vi "CLD 15 Address Parsing SubVI.vi"(8 "Fehler (Eingang)":errorcluster, 10 "Daten-String (Eingang)":string, 11 "Datenstruktur der CSV-Datei (Eingang)":T1) -> (0 "Fehler (Ausgang)":errorcluster, 3 "Datenstruktur der CSV-Datei (Ausgang)":T1)   [LabVIEW 2009]
doc: "CLD 15 - Analyseroutine für den Adress-String in CLD 15. Dieser String enthält auch den Rabatt in Prozent. Die Preise und der Schwellwert für eine Großbestellung werden der Spezifikation entnommen.\n\nDie Datenformate werden der Spezifikation als freie Beschriftungen entnommen, um zu vermeiden, dass sie während der Programmierung erneut geprüft werden."
uses:
  CLD 15 CSV file data structure.ctl
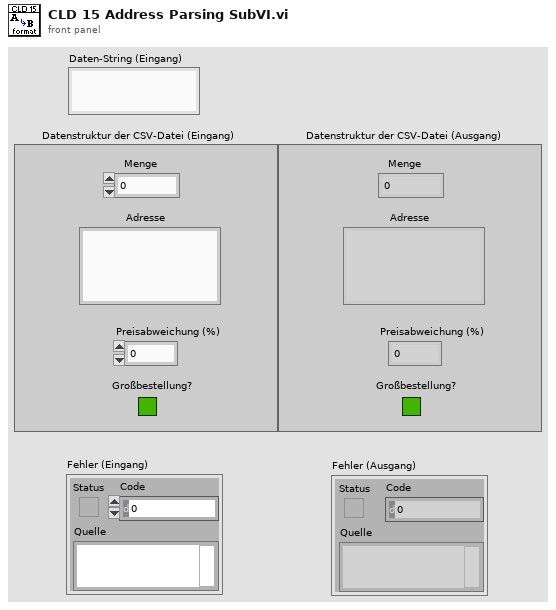
[diagram p1: front panel]
types:
  T1 = typedef "CLD 15 CSV file data structure.ctl" = cluster{"Menge":i32, "Adresse":string, "Preisabweichung (%)":dbl, "Großbestellung?":bool}
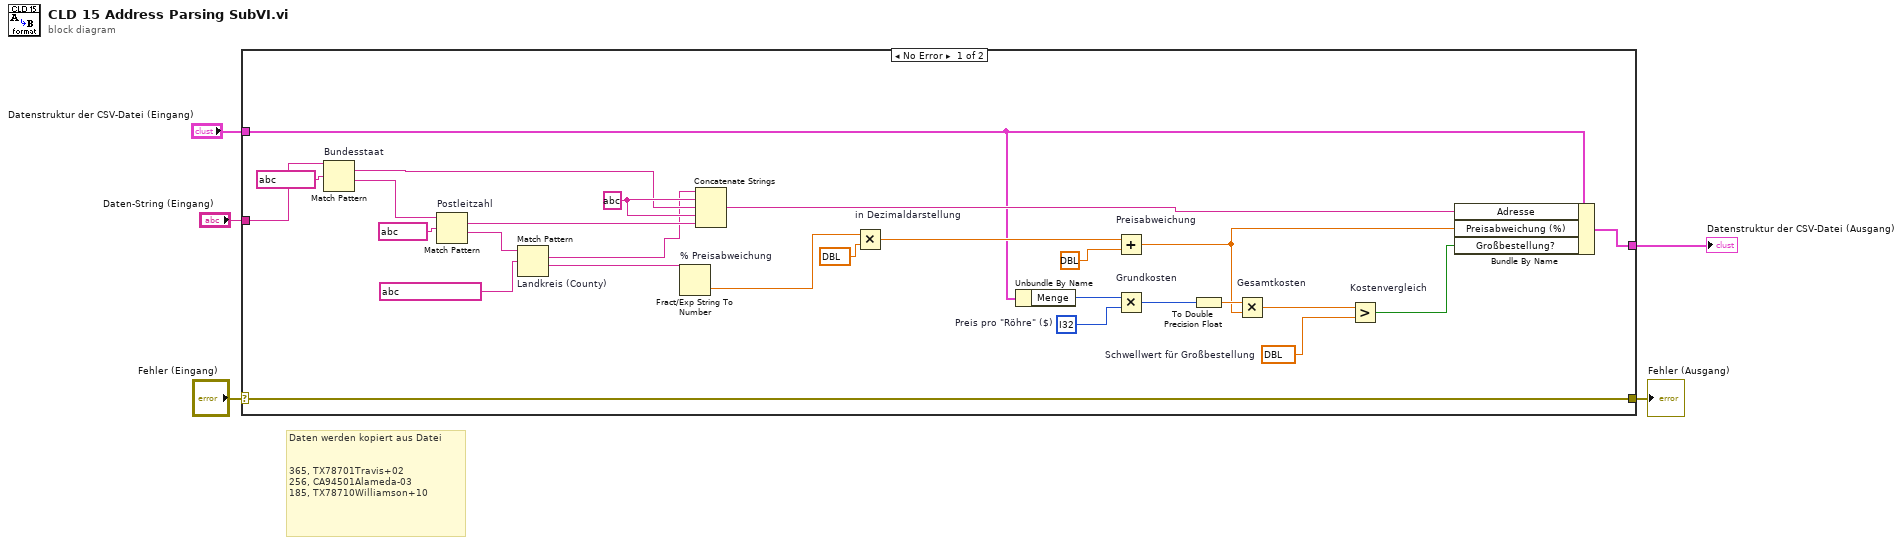
[diagram p0: block diagram]
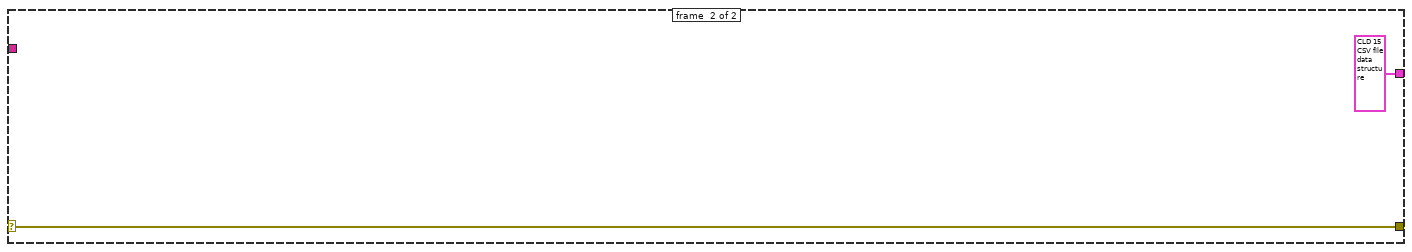
[diagram p2: hidden frame]
diagram:
  # "Daten werden kopiert aus Datei\n\n\n365,\tTX78701Travis+02\n256,\tCA94501Alameda-03\n185,\tTX78710Williamson+10"
  n1 = case shown="No Error" "Fehler (Eingang)" {
    selector: "Fehler (Eingang)" -> [w7 w34]
    tunnel: [w32 T1 ? ("Datenstruktur der CSV-Datei (Eingang)")] -> w5
    tunnel: "Daten-String (Eingang)" -> [w31 _]
    tunnel: [w7 w34] -> w2
    tunnel: "Datenstruktur der CSV-Datei (Eingang)" -> [w6 _]
    frame #0 {
      w14 = dbl ?  # Schwellwert für Großbestellung
      w19 = i32 ?  # Preis pro "Röhre" ($)
      w29 = string ?
      n2 = Match Pattern "Bundesstaat"(string=w31, regular expression=string ?) -> (match substring=w28:string, after substring=w27:string)  [unwired: 1 in, 2 out]
      n3 = Match Pattern "Postleitzahl"(string=w27, regular expression=string ?) -> (match substring=w25:string, after substring=w24:string)  [unwired: 1 in, 2 out]
      n4 = Match Pattern "Landkreis (County)"(string=w24, regular expression=string ?) -> (match substring=w23:string, after substring=w21:string)  [unwired: 1 in, 2 out]
      n5 = Fract/Exp String To Number "% Preisabweichung"(string=w21) -> (number=w9:dbl)  [unwired: 3 in, 1 out]
      n6 = Concatenate Strings(w23, w29, w28, w29, w25) -> (w22:string)
      n7 = Multiply "in Dezimaldarstellung"(x=w9, y=dbl ?) -> (x*y=w8:dbl)
      n8 = Unbundle By Name(w6) -> ("Menge"=w20:i32)
      n9 = Add "Preisabweichung"(x=w8, y=dbl ?) -> (x+y=w11:dbl)
      n10 = Multiply "Grundkosten"(x=w20, y=w19) -> (x*y=w17:i32)
      n11 = To Double Precision Float(number=w17) -> (double precision float=w16:dbl)
      n12 = Multiply "Gesamtkosten"(x=w16, y=w11) -> (x*y=w15:dbl)
      n13 = Greater? "Kostenvergleich"(x=w15, y=w14) -> (0:w13:bool)
      n14 = Bundle By Name(cluster=w6, "Adresse"=w22, "Preisabweichung (%)"=w11, "Großbestellung?"=w13) -> (w32:T1)
    }
    frame #1 {
    }
  }
  "Datenstruktur der CSV-Datei (Ausgang)" <- w5
  "Fehler (Ausgang)" <- w2
